vi "parseMotionStatusShortStatus.vi"(8 "error in (no error)":errorcluster, 10 "shortStatus":string, 11 "DomeCommunicator in":refnum<class "DomeCommunicator.lvclass">) -> (0 "error out":errorcluster, 1 "state":T1, 2 "LastRotationDirection":T4, 3 "DomeCommunicator out":refnum<class "DomeCommunicator.lvclass">)   [LabVIEW 2016, in "DomeCommunicator.lvclass"]
uses:
  DomeCommunicator.lvclass
  IDome/domeTypedefs/direction.ctl
  IDome/domeTypedefs/domeState.ctl
  IDome/domeTypedefs/motionDirection.ctl
  IDome/domeTypedefs/openingMotion.ctl
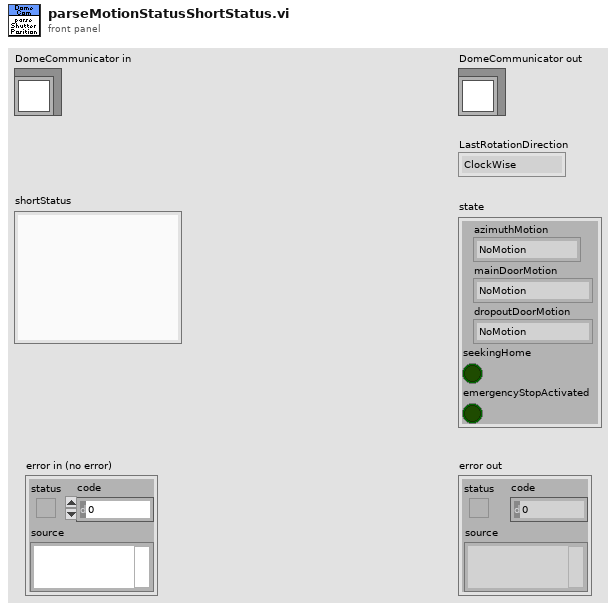
[diagram p1: front panel]
types:
  T1 = typedef "domeState.ctl" = cluster{"azimuthMotion":T2, "mainDoorMotion":T3, "dropoutDoorMotion ":T3, "seekingHome":bool, "emergencyStopActivated":bool}
  T2 = typedef "motionDirection.ctl" = enum16{"NoMotion", "MovingClockWise", "MovingCounterClockWise"}
  T3 = typedef "openingMotion.ctl" = enum16{"NoMotion", "Opening", "Closing"}
  T4 = typedef "direction.ctl" = enum16{"ClockWise", "CounterClockWise"}
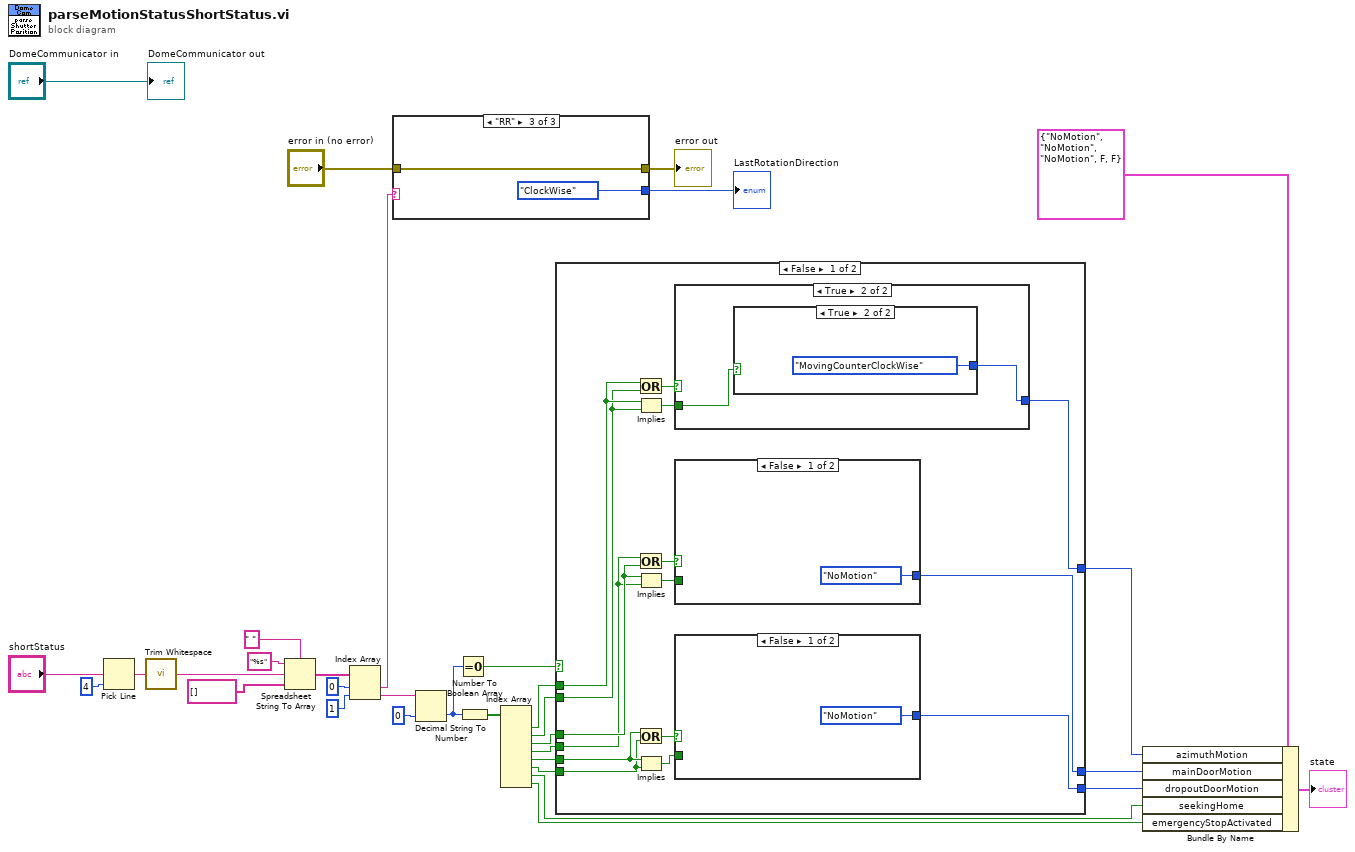
[diagram p0: block diagram]
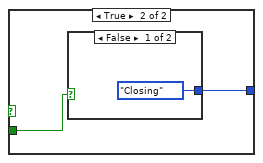
[diagram p2: hidden frame]
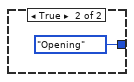
[diagram p3: hidden frame]
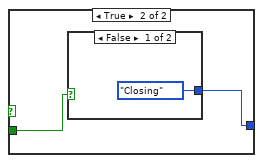
[diagram p4: hidden frame]
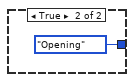
[diagram p5: hidden frame]
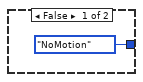
[diagram p6: hidden frame]
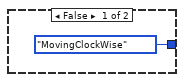
[diagram p7: hidden frame]
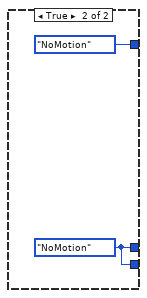
[diagram p8: hidden frame]
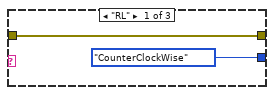
[diagram p9: hidden frame]
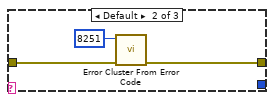
[diagram p10: hidden frame]
diagram:
  n1 = Pick Line(multi-line string="shortStatus", line index=4) -> (output string=w31:string)  [unwired: 1 in]
  n2 = call <vilib>:"Trim Whitespace.vi"("string"=w31) -> ("trimmed string"=w26:string)  [unwired: 1 in]
  n3 = Spreadsheet String To Array(delimiter (Tab)=" ", format string="%s", spreadsheet string=w26, array type (2D Dbl)=string[] []) -> (array=w22:string[])
  n4 = Index Array(array=w22, index #1=0 ("index"), index #2=1 ("index")) -> (element #1=w20:string, element #2=w15:string)
  n5 = case shown="\"RR\"" w20 {
    tunnel: "error in (no error)" -> [w35 w37 w40]
    tunnel: [w35 w38 w40] -> w25
    tunnel: [direction."CounterClockWise" ("LastRotationDirection") _ direction."ClockWise" ("LastRotationDirection")] -> w19
    frame "RL" {
    }
    frame Default {
      n6 = call <vilib>:"Error Cluster From Error Code.vi"("error in (no error)"=w37, "error code (0)"=8251) -> ("error out"=w38:errorcluster)  [unwired: 7 in]
    }
    frame "RR" {
    }
  }
  "error out" <- w25
  "LastRotationDirection" <- w19
  n7 = Decimal String To Number(string=w15, default (0L)=u16 0) -> (number=w8:u16)  [unwired: 1 in, 1 out]
  n8 = Equal To 0?(x=w8) -> (x = 0?=w7:bool)
  n9 = Number To Boolean Array(number=w8) -> (Boolean array=w14:bool[])
  n10 = Index Array(array=w14) -> (element #1=w6:bool, element #2=w5:bool, element #3=w4:bool, element #4=w3:bool, element #5=w2:bool, element #6=w1:bool, element #7=w12:bool, element #8=w13:bool)  [unwired: 8 in]
  n11 = case shown="False" w7 {
    tunnel: [w52 motionDirection."NoMotion" ("azimuthMotion")] -> w11
    tunnel: [w51 w71] -> w10
    tunnel: [w50 w71] -> w9
    tunnel: w6 -> [w49 _]
    tunnel: w5 -> [w48 _]
    tunnel: w4 -> [w45 _]
    tunnel: w3 -> [w44 _]
    tunnel: w2 -> [w42 _]
    tunnel: w1 -> [w41 _]
    frame False {
      n12 = Or(x=w49, y=w48) -> (x .or. y?=w47:bool)
      n13 = Implies(1:w48, 2:w49) -> (0:w53:bool)
      n14 = Or(x=w44, y=w45) -> (x .or. y?=w46:bool)
      n15 = Implies(1:w44, 2:w45) -> (0:w54:bool)
      n16 = Or(x=w42, y=w41) -> (x .or. y?=w43:bool)
      n17 = Implies(1:w41, 2:w42) -> (0:w55:bool)
      n18 = case shown="True" w47 {
        tunnel: w53 -> [_ w68]
        tunnel: [motionDirection."NoMotion" ("azimuthMotion") w67] -> w52
        frame False {
        }
        frame True {
          n19 = case shown="True" w68 {
            tunnel: [motionDirection."MovingClockWise" ("azimuthMotion") motionDirection."MovingCounterClockWise" ("azimuthMotion")] -> w67
            frame False {
            }
            frame True {
            }
          }
        }
      }
      n20 = case shown="False" w46 {
        tunnel: w54 -> [_ w63]
        tunnel: [openingMotion."NoMotion" ("mainDoorMotion") w62] -> w51
        frame False {
        }
        frame True {
          n21 = case shown="False" w63 {
            tunnel: [openingMotion."Closing" ("mainDoorMotion") openingMotion."Opening" ("mainDoorMotion")] -> w62
            frame False {
            }
            frame True {
            }
          }
        }
      }
      n22 = case shown="False" w43 {
        tunnel: w55 -> [_ w58]
        tunnel: [openingMotion."NoMotion" ("mainDoorMotion") w57] -> w50
        frame False {
        }
        frame True {
          n23 = case shown="False" w58 {
            tunnel: [openingMotion."Closing" ("mainDoorMotion") openingMotion."Opening" ("mainDoorMotion")] -> w57
            frame False {
            }
            frame True {
            }
          }
        }
      }
    }
    frame True {
      w71 = openingMotion."NoMotion" ("mainDoorMotion")
    }
  }
  n24 = Bundle By Name(cluster=T1 {"azimuthMotion"=enum."NoMotion", "mainDoorMotion"=enum."NoMotion", "dropoutDoorMotion "=enum."NoMotion", "seekingHome"=FALSE, "emergencyStopActivated"=FALSE} ("state"), "azimuthMotion"=w11, "mainDoorMotion"=w10, "dropoutDoorMotion"=w9, "seekingHome"=w12, "emergencyStopActivated"=w13) -> (→"state":T1)
  "DomeCommunicator out" <- "DomeCommunicator in"
